vi "configure.vi"(8 "error in (no error)":errorcluster, 11 "GenericPlugin in":refnum<class "ComponentTemplate.lvclass">) -> (0 "error out":errorcluster, 3 "GenericPlugin out":refnum<class "ComponentTemplate.lvclass">)   [LabVIEW 2010]
doc: "The dynamic dispatch version of this VI loads and displays the configuration file associated with the plug-in object. The user modify and save the configuration data."
uses:
  common/classes/GenericComponent/GenericComponent/GenericComponent.lvclass
  ComponentTemplate.lvclass
panel:
  out "configuration":string
  in  "cancelButton":bool
  in  "okButton":bool
  # "Configure XY"
  # "1. Put controls for your configuration values here and their value change events in the event structure on the block diagram."
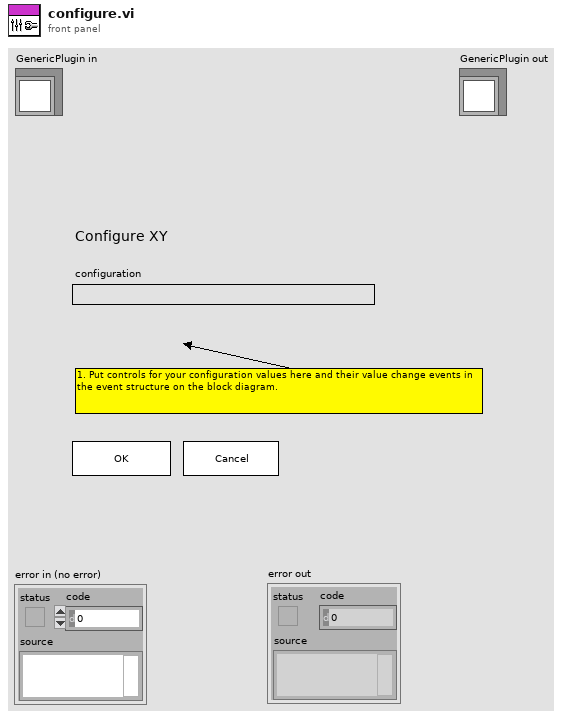
[diagram p1: front panel]
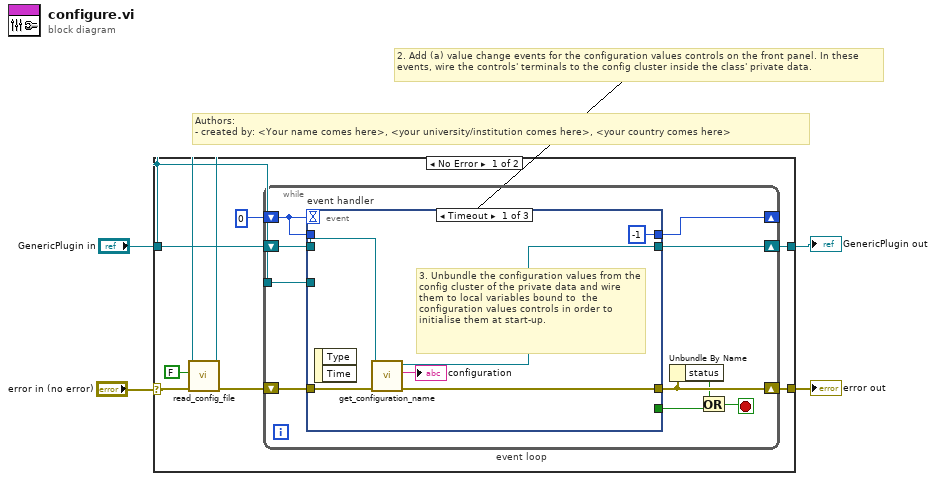
[diagram p0: block diagram]
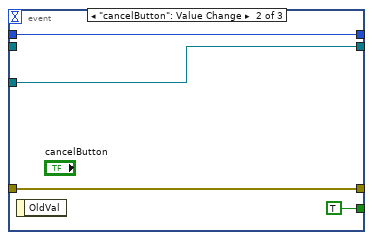
[diagram p2: hidden frame]
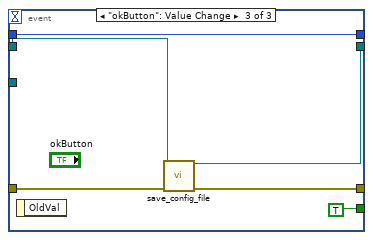
[diagram p3: hidden frame]
diagram:
  # "2. Add (a) value change events for the configuration values controls on the front panel. In these events, wire the controls' terminals to the config cluster inside the class' private data."
  # "Authors: \n- created by: <Your name comes here>, <your university/institution comes here>, <your country comes here>"
  n1 = case shown="No Error" "error in (no error)" {
    selector: "error in (no error)" -> [w9 w38]
    tunnel: [w11 w38] -> w3
    tunnel: "GenericPlugin in" -> [w7 w39]
    tunnel: [w10 w39] -> w1
    frame No Error {
      n2 = call-dynamic "read_config_file.vi"("GenericPlugin out"=w7, "error in (no error)"=w9, "force load?"=FALSE, "GenericPlugin in"=w7) -> ("error out"=w8:errorcluster)  [unwired: 7 in]
      n3 = while "event loop" {
        shift-right: [w18] -> w11
        shift-left: w8 -> [w21]
        shift-right: [w19] -> w10
        shift-left: w7 -> [w20]
        tunnel: w7 -> [w14]
        shift-right: [w12] -> _
        shift-left: 0 -> [w13]
        stop <- w15 stop-if-true
        n4 = event "event handler" shown="[0] Timeout" {
          selector: _ -> [_ _ _]
          dyn-events: _ -> [_ _ _]
          timeout: w13 -> [_ _ _]
          tunnel: w21 -> [w27 w31 w36]
          tunnel: [w26 w31 w35] -> w18
          tunnel: w20 -> [w25 _ w34]
          tunnel: [w24 w29 w33] -> w19
          tunnel: [_ TRUE TRUE] -> w17
          tunnel: w14 -> [_ w29 _]
          tunnel: [-1 w28 w32] -> w12
          tunnel: w13 -> [_ w28 w32]
          event Timeout {
            # "3. Unbundle the configuration values from the config cluster of the private data and wire them to local variables bound to  the configuration values controls in order to initialise them at start-up."
            n5 = event-data() -> ()  [unwired: 1 in, 2 out]
            n6 = call "get_configuration_name.vi"("error in (no error)"=w27, "GenericPlugin.lvclass in"=w25) -> ("error out"=w26:errorcluster, "configuration name"=→"configuration":string, "GenericPlugin.lvclass out"=w24:refnum<class "GenericComponent.lvclass">)  [unwired: 7 in]
          }
          event "cancelButton": Value Change {
            n7 = event-data() -> ()  [unwired: 1 in, 1 out]
          }
          event "okButton": Value Change {
            n8 = event-data() -> ()  [unwired: 1 in, 1 out]
            n9 = call-dynamic "save_config_file.vi"("error in (no error)"=w36, "GenericPlugin in"=w34) -> ("error out"=w35:errorcluster, "GenericPlugin out"=w33:refnum<class "GenericComponent.lvclass">)  [unwired: 8 in]
          }
        }
        n10 = Unbundle By Name(w18) -> ("status"=w16:bool)
        n11 = Or(x=w16, y=w17) -> (x .or. y?=w15:bool)
      }
    }
    frame Error {
    }
  }
  "error out" <- w3
  "GenericPlugin out" <- w1
